vi "Init Record File.vi"() -> (3 "Byte Stream File out":refnum<file>)   [LabVIEW 2015]
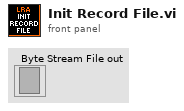
[diagram p1: front panel]
types:
  T1 = enum16{"open", "replace", "create", "open or create", "replace or create", "replace or create with confirmation"}
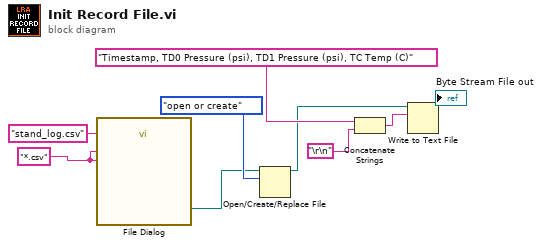
[diagram p0: block diagram]
diagram:
  w1 = "*.csv" ("pattern label")
  n1 = call "File Dialog"("default name"="stand_log.csv", "pattern (all files)"=w1, "pattern label"=w1) -> ("selected path"=w3:path)  [unwired: 9 in, 3 out]
  n2 = Open/Create/Replace File(file path (use dialog)=w3, operation (0:open)=T1."open or create") -> (refnum out=w5:refnum<file>)  [unwired: 4 in, 2 out]
  n3 = Concatenate Strings("Timestamp, TD0 Pressure (psi), TD1 Pressure (psi), TC Temp (C)" ("text"), "\r\n") -> (w9:string)
  n4 = Write to Text File(file (use dialog)=w5, text=w9) -> (refnum out=→"Byte Stream File out":refnum<file>)  [unwired: 2 in, 2 out]
